vi "Send_Init_States.vi"(7 "Filename (.ini)":string="Config_Ver_1\\pulse_sequence.ini", 8 "error in":errorcluster, 11 "VISA arduino in":refnum<visa-resource-name>) -> (0 "error out":errorcluster, 1 "register 2 (8-13)":T1, 2 "register 1 (2-7)":T2, 3 "VISA arduino out":refnum<visa-resource-name>)   [LabVIEW 2021]
uses:
  Drivers/Arduino_Pulse_Generator/Configurate/Register_1.ctl
  Drivers/Arduino_Pulse_Generator/Configurate/Register_2.ctl
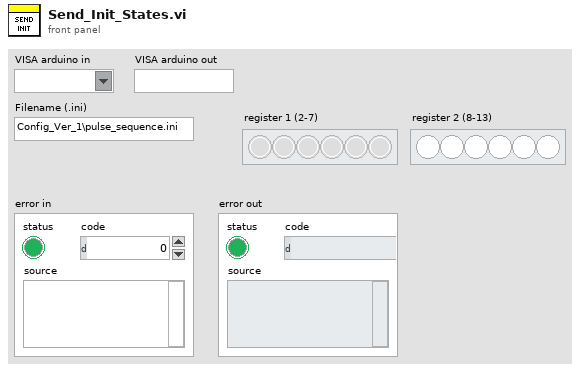
[diagram p1: front panel]
types:
  T1 = typedef "Register_2.ctl" = bool[]
  T2 = typedef "Register_1.ctl" = bool[]
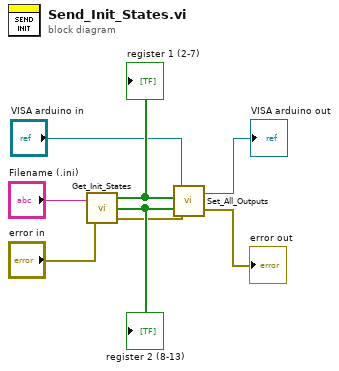
[diagram p0: block diagram]
diagram:
  n1 = call "Get_Init_States.vi"("Filename (.ini)"="Filename (.ini)", "error in"="error in") -> ("register 1 (2-7)"=w8:T2, "register 2 (8-13)"=w7:T1, "error out"=w6:errorcluster)
  "register 1 (2-7)" <- w8
  "register 2 (8-13)" <- w7
  n2 = call "Set_All_Outputs.vi"("error in"=w6, "register 2 (8-13)"=w7, "register 1 (2-7)"=w8, "VISA arduino in"="VISA arduino in") -> ("error out"=→"error out":errorcluster, "VISA arduino out"=→"VISA arduino out":refnum<visa-resource-name>)
